vi "getChannelStates.vi"(8 "error in (no error)":errorcluster, 11 "ScriptEvent in":refnum<class "ScriptEvent.lvclass">) -> (0 "error out":errorcluster, 2 "statesValues":string[](array[string]), 3 "ScriptEvent out":refnum<class "ScriptEvent.lvclass">)   [LabVIEW 2011, in "Tools.lvlib" / "Scripting.lvlib" / "ScriptEvent.lvclass"]
uses:
  ScriptEvent.lvclass
  ScriptEvent.lvclass/ScriptEvent.ctl
  DatabaseHelpers/Database Objects/Channel/Channel.lvclass
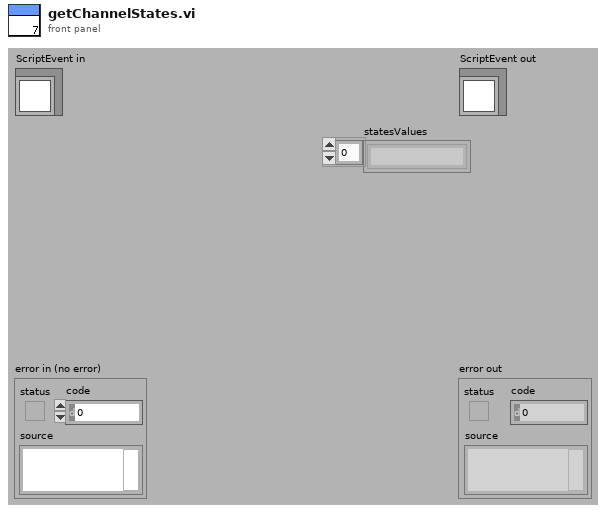
[diagram p1: front panel]
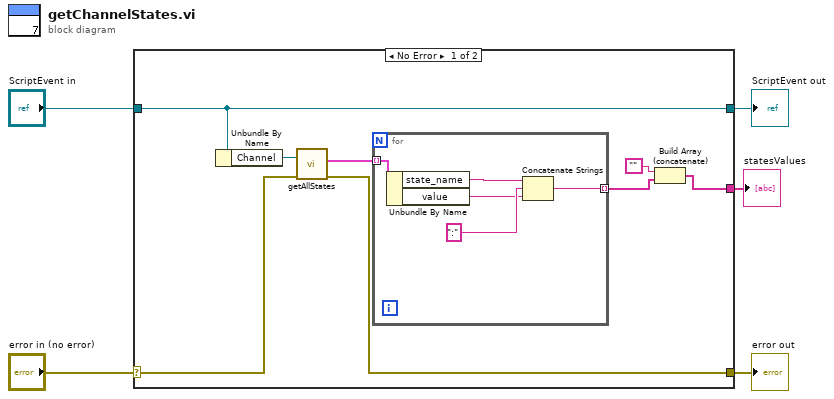
[diagram p0: block diagram]
diagram:
  n1 = case shown="No Error" "error in (no error)" {
    selector: "error in (no error)" -> [w11 w20]
    tunnel: [w9 w20] -> w4
    tunnel: [w13 w19] -> w2
    tunnel: "ScriptEvent in" -> [w13 w19]
    tunnel: [w7 _] -> w1
    frame No Error {
      n2 = Unbundle By Name(w13) -> ("Channel"=w12:refnum<class "Channel.lvclass">)
      n3 = call "getAllStates.vi"("error in (no error)"=w11, "Channel.lvclass in"=w12) -> ("error out"=w9:errorcluster, "states"=w10:cluster{"state_name":string, "value":string}[])  [unwired: 7 in, 1 out]
      n4 = for {
        tunnel: w10 -> [w18] mode=indexing
        tunnel: [w14] -> w8 mode=indexing
        n5 = Unbundle By Name(w18) -> ("state_name"=w17:string, "value"=w15:string)
        n6 = Concatenate Strings(w17, ":", w15) -> (w14:string)
      }
      n7 = Build Array (concatenate)("", w8) -> (w7:string[])
    }
    frame Error {
    }
  }
  "error out" <- w4
  "ScriptEvent out" <- w2
  "statesValues" <- w1
